vi "Drop Message.vi"(11 "Message in":refnum<class "Message.lvclass">) -> ()   [LabVIEW 2017, in "Actor Framework.lvlib" / "Message.lvclass"]
doc: "(<B>Filename</B>: Actor Framework.lvlib:Message.lvclass:Drop Message.vi)\n\nWrapper for Drop Message Core.vi"
uses:
  <vilib>/ActorFramework/Message/Message.lvclass
  <resource>/AFDebug/AF Debug.lvlib
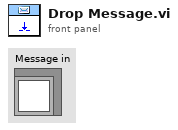
[diagram p1: front panel]
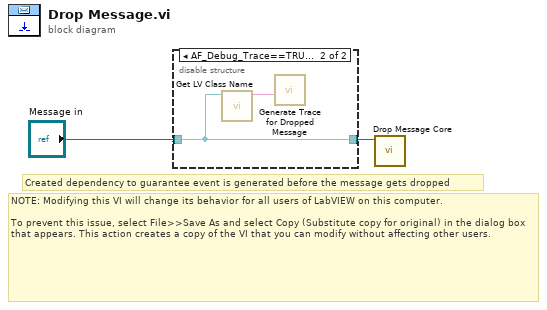
[diagram p0: block diagram]
diagram:
  # "Created dependency to guarantee event is generated before the message gets dropped"
  # "NOTE: Modifying this VI will change its behavior for all users of LabVIEW on this computer.\n\nTo prevent this issue, select File>>Save As and select Copy (Substitute copy for original) in the dialog box that appears. This action creates a copy of the VI that you can modify without affecting other users."
  n1 = disable-structure shown="AF_Debug_Trace==TRUE" {
    disable-tunnel: "Message in" -> [w3 w4]
    disable-tunnel: [w3 w4] -> w1
    frame condition #0 (active) {
    }
    frame condition #1 {
      n2 = call <vilib>:"Get LV Class Name.vi"("object"=w4) -> ("class name"=w5:string)  [unwired: 9 in, 1 out]
      n3 = call <resource>:"Generate Trace for Dropped Message.vi"("Message Name"=w5) -> ()  [unwired: 11 in]
    }
  }
  n4 = call-dynamic "Drop Message Core.vi"("Message in"=w1) -> ()  [unwired: 11 in]
